vi "db.vi"(6 "Gen SN?":bool, 7 "DB File":path=path "D:/Valeo/Micriphone Test/UI/data.s3db", 8 "error in (no error)":errorcluster, 10 "Datas In":dbl[](array[numeric]), 11 "Model":string="ME79") -> (0 "error out":errorcluster, 1 "SN Out":string, 2 "Last INSERT RowID":i64)   [LabVIEW 2018]
uses:
  <vilib>/drjdpowell/SQLite Library/SQL Connection/Connection.lvclass/Connection.ctl
  <vilib>/drjdpowell/SQLite Library/SQL Connection/Open (path).vi
  <vilib>/drjdpowell/SQLite Library/SQL Connection/Open (string).vi
  <vilib>/AdvancedString/Path To Command Line String.vi
  <vilib>/drjdpowell/SQLite Library/SQL Connection/Execute SQL (Single Integer).vi
  <vilib>/drjdpowell/SQLite Library/SQL Connection/Execute SQL (No results).vi
  <vilib>/drjdpowell/SQLite Library/SQL Connection/Connection.lvclass
  <vilib>/drjdpowell/SQLite Library/SQLite.lvlib
panel:
  out "Last SN":i64
  out "date/time string":string
  out "sql":string
  out "Model Id":i64
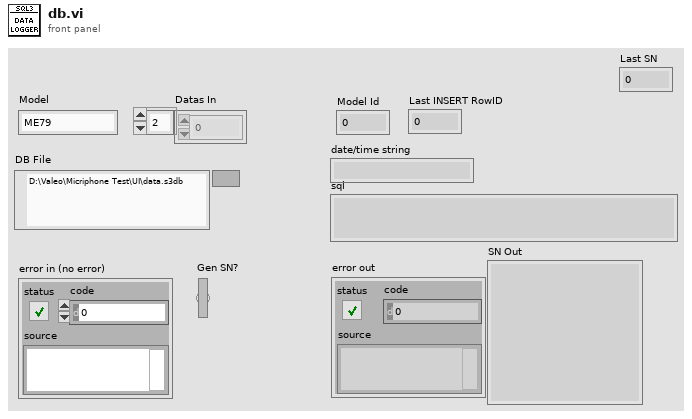
[diagram p1: front panel]
types:
  T1 = enum16{"New or existing", "Existing", "Read only"}
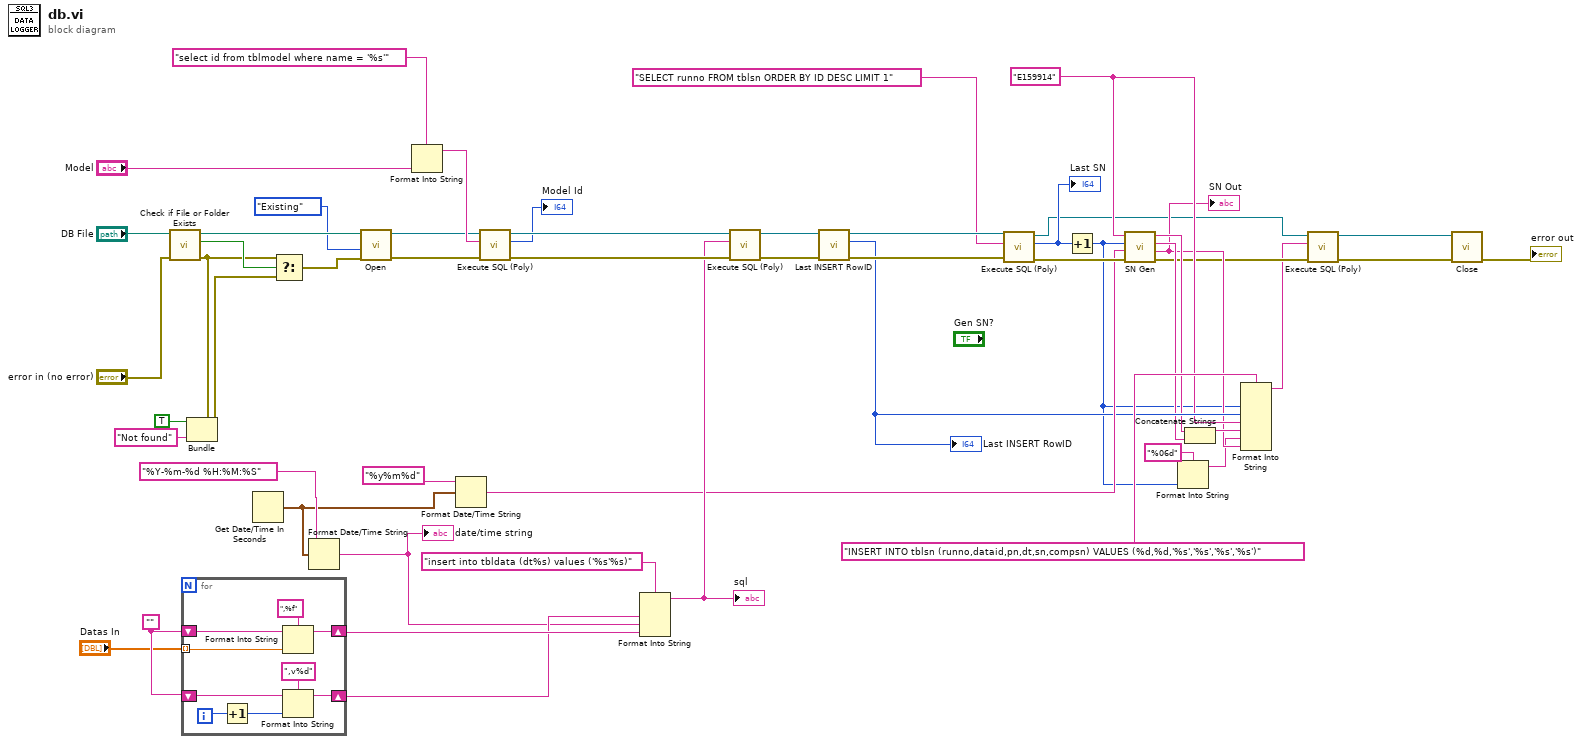
[diagram p0: block diagram]
diagram:
  w12 = "E159914" ("PN In")
  w32 = ""
  n1 = call <vilib>:"Check if File or Folder Exists.vi"("error in (no error)"="error in (no error)", "path"="DB File") -> ("error out"=w46:errorcluster, "file or folder exists?"=w47:bool, "dup path"=w44:path)  [unwired: 7 in]
  n2 = for {
    tunnel: "Datas In" -> [w60] mode=indexing
    shift-right: [w55] -> w36
    shift-left: w32 -> [w52]
    shift-right: [w54] -> w35
    shift-left: w32 -> [w53]
    i -> [w59]
    n3 = Increment(x=w59) -> (x+1=w58:i32)
    n4 = Format Into String(format string=",%f", initial string=w52, w60) -> (resulting string=w55:string)  [unwired: 1 in, 1 out]
    n5 = Format Into String(format string=",v%d", initial string=w53, w58) -> (resulting string=w54:string)  [unwired: 1 in, 1 out]
  }
  n6 = Bundle(cluster=w46, "status"=TRUE, "source"="Not found") -> (w45:errorcluster)  [unwired: 1 in]
  n7 = Get Date/Time In Seconds() -> (seconds since 1Jan1904=w17:timestamp)
  n8 = Select(t=w46, s=w47, f=w45) -> (s? t:f=w42:errorcluster)
  n9 = Format Date/Time String(time format string (%c)="%Y-%m-%d %H:%M:%S", seconds (now)=w17) -> (date/time string=w34:string)  [unwired: 1 in]
  "date/time string" <- w34
  n10 = call-poly <vilib>:"Open.vi"("error in (no error)"=w42, "File Option"=T1."Existing", "db file"=w44) -> ("error out"=w39:errorcluster, "SQLite Connection"=w38:refnum<class "Connection.lvclass">)  [unwired: 7 in]
  n11 = Format Into String(format string="select id from tblmodel where name = '%s'", "Model") -> (resulting string=w40:string)  [unwired: 2 in, 1 out]
  n12 = Format Date/Time String(time format string (%c)="%y%m%d", seconds (now)=w17) -> (date/time string=w15:string)  [unwired: 1 in]
  n13 = call-poly <vilib>:"Execute SQL (Poly).vi"("error in (no error)"=w39, "SQL"=w40, "SQLite Connection in"=w38) -> ("error out"=w28:errorcluster, "Result"=→"Model Id":i64, "SQLite Connection"=w29:refnum<class "Connection.lvclass">)  [unwired: 6 in]
  n14 = Format Into String(format string="insert into tbldata (dt%s) values ('%s'%s)", w35, w34, w36) -> (resulting string=w27:string)  [unwired: 2 in, 1 out]
  "sql" <- w27
  n15 = call-poly <vilib>:"Execute SQL (Poly).vi"("error in (no error)"=w28, "SQL"=w27, "SQLite Connection in"=w29) -> ("error out"=w23:errorcluster, "SQLite Connection"=w24:refnum<class "Connection.lvclass">)  [unwired: 7 in]
  n16 = call <vilib>:"Last INSERT RowID.vi"("error in (no error)"=w23, "SQLite Connection in"=w24) -> ("error out"=w21:errorcluster, "Last INSERT RowID"=w13:i64, "SQLite Connection"=w22:refnum<class "Connection.lvclass">)  [unwired: 7 in]
  "Last INSERT RowID" <- w13
  n17 = call-poly <vilib>:"Execute SQL (Poly).vi"("error in (no error)"=w21, "SQL"="SELECT runno FROM tblsn ORDER BY ID DESC LIMIT 1", "SQLite Connection in"=w22) -> ("error out"=w16:errorcluster, "Result"=w19:i64, "SQLite Connection"=w2:refnum<class "Connection.lvclass">)  [unwired: 6 in]
  "Last SN" <- w19
  n18 = Increment(x=w19) -> (x+1=w5:i64)
  n19 = call "SN Gen.vi"("error in (no error)"=w16, "Date In"=w15, "SN In"=w5, "PN In"=w12) -> ("error out"=w4:errorcluster, "SN Out"=w8:string, "Shift"=w11:string, "Date"=w10:string)  [unwired: 4 in]
  "SN Out" <- w8
  n20 = Format Into String(format string="%06d", w5) -> (resulting string=w7:string)  [unwired: 2 in, 1 out]
  n21 = Concatenate Strings(w10, w11) -> (w9:string)
  n22 = Format Into String(format string="INSERT INTO tblsn (runno,dataid,pn,dt,sn,compsn) VALUES (%d,%d,'%s','%s','%s','%s')", w5, w13, w12, w9, w7, w8) -> (resulting string=w3:string)  [unwired: 2 in, 1 out]
  n23 = call-poly <vilib>:"Execute SQL (Poly).vi"("error in (no error)"=w4, "SQL"=w3, "SQLite Connection in"=w2) -> ("SQLite Connection"=w1:refnum<class "Connection.lvclass">)  [unwired: 7 in, 1 out]
  n24 = call-dynamic "Close.vi"("error in (no error)"=w4, "SQLite Connection in"=w1) -> ("error out"=→"error out":errorcluster)  [unwired: 9 in]
